vi "Sub03_PosTxt.vi"(8 "error in (no error)":errorcluster, 10 "String":string) -> (0 "error out":errorcluster, 3 "output cluster":T1, 5 "standard error":string, 7 "standard output":string)   [LabVIEW 2019]
panel:
  out "vi name":string
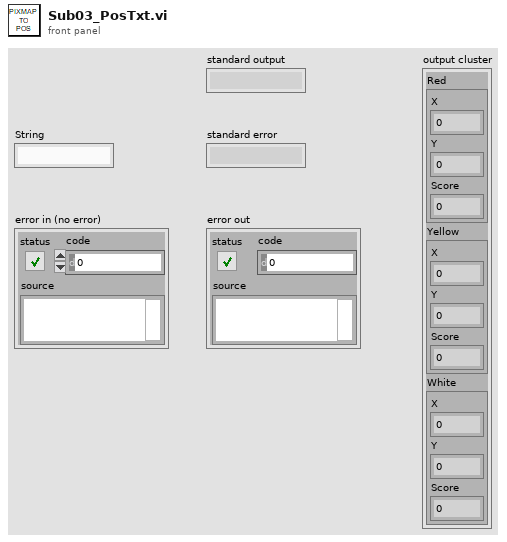
[diagram p1: front panel]
types:
  T1 = cluster{"Red":cluster{"X":u32, "Y":u32, "Score":u32}, "Yellow":cluster{"X":u32, "Y":u32, "Score":u32}, "White":cluster{"X":u32, "Y":u32, "Score":u32}}
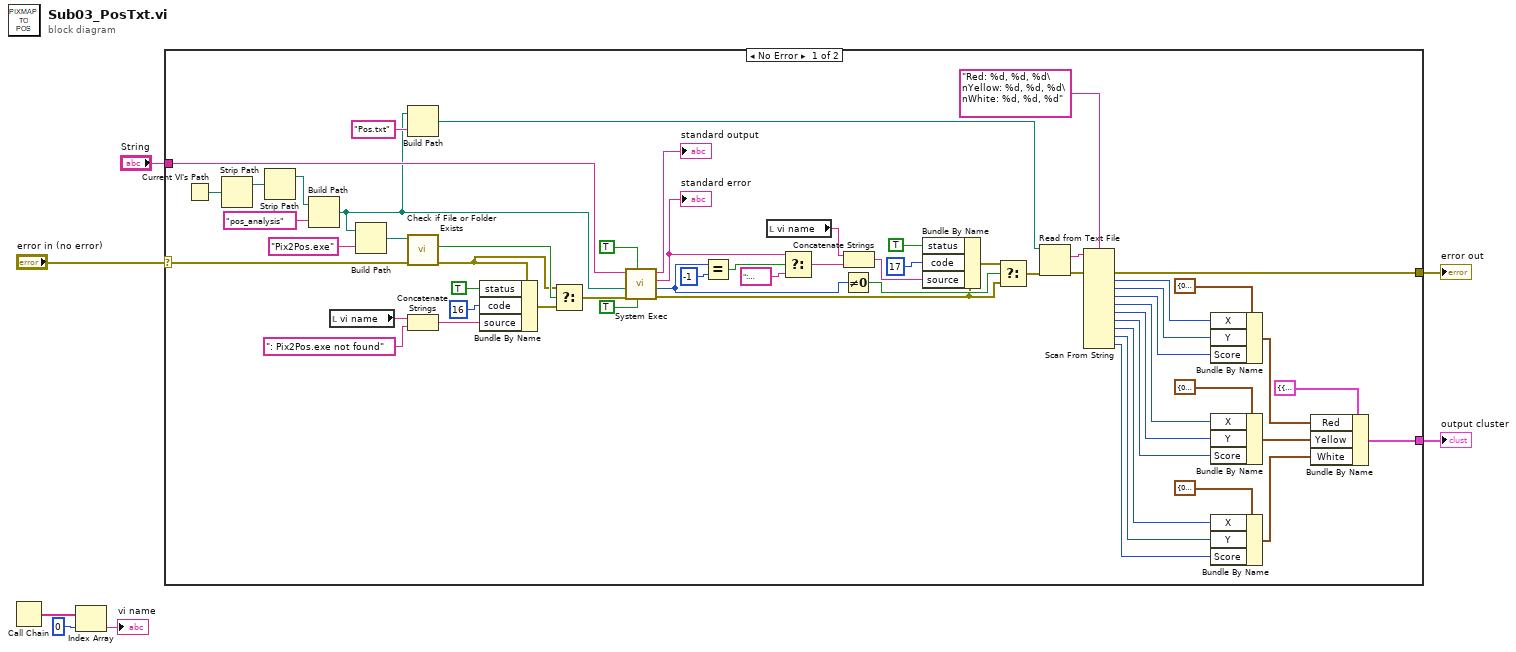
[diagram p0: block diagram]
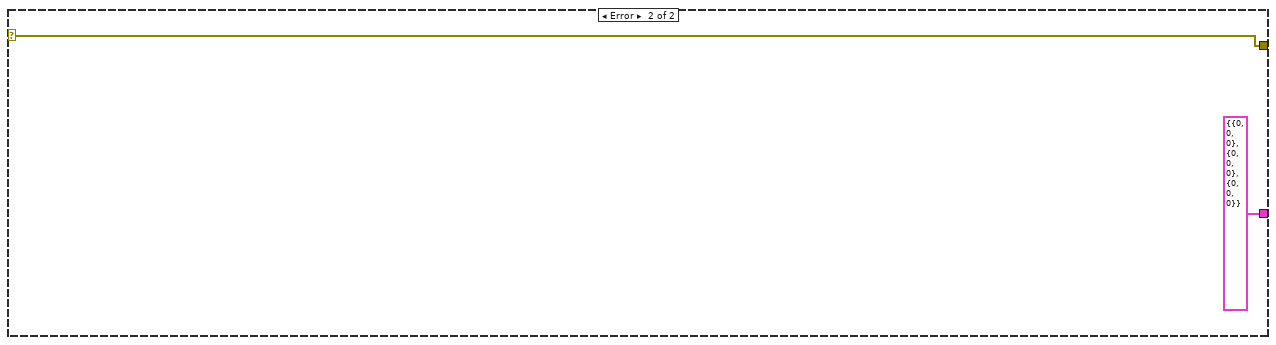
[diagram p2: hidden frame]
diagram:
  n1 = Call Chain() -> (call chain=w3:string[])
  n2 = Index Array(array=w3, index=0) -> (element=→"vi name":string)
  n3 = case shown="No Error" "error in (no error)" {
    selector: "error in (no error)" -> [w23 w66]
    tunnel: [w29 w66] -> w7
    tunnel: [w28 T1 {"Red"={"X"=0, "Y"=0, "Score"=0}, "Yellow"={"X"=0, "Y"=0, "Score"=0}, "White"={"X"=0, "Y"=0, "Score"=0}} ("output cluster")] -> w6
    tunnel: "String" -> [w27 _]
    frame No Error {
      n4 = Current VI's Path() -> (path=w30:path)
      n5 = Strip Path(path=w30) -> (stripped path=w11:path)  [unwired: 1 out]
      n6 = Strip Path(path=w11) -> (stripped path=w10:path)  [unwired: 1 out]
      n7 = Build Path(base path=w10, name or relative path="pos_analysis") -> (appended path=w9:path)
      n8 = local read "vi name"() -> (w13:string)
      n9 = Build Path(base path=w9, name or relative path="Pix2Pos.exe") -> (appended path=w26:path)
      n10 = Build Path(base path=w9, name or relative path="Pos.txt") -> (appended path=w60:path)
      n11 = call <vilib>:"Check if File or Folder Exists.vi"("error in (no error)"=w23, "path"=w26) -> ("error out"=w16:errorcluster, "file or folder exists?"=w24:bool)  [unwired: 7 in, 1 out]
      n12 = Concatenate Strings(w13, ": Pix2Pos.exe not found" ("string")) -> (w18:string)
      n13 = Bundle By Name(cluster=w16, "status"=TRUE, "code"=16, "source"=w18) -> (w17:errorcluster)
      n14 = Select(t=w16, s=w24, f=w17) -> (s? t:f=w22:errorcluster)
      n15 = call <vilib>:"System Exec.vi"("run minimized? (F)"=TRUE, "wait until completion? (T)"=TRUE, "error in (no error)"=w22, "working directory"=w9, "command line"=w27) -> ("error out"=w31:errorcluster, "return code"=w35:i32, "standard error"=w33:string, "standard output"=→"standard output":string)  [unwired: 3 in]
      "standard error" <- w33
      n16 = Equal?(x=w35, y=-1) -> (x = y?=w36:bool)
      n17 = local read "vi name"() -> (w12:string)
      n18 = Select(t=w33, s=w36, f=": unknown error during C execution") -> (s? t:f=w15:string)
      n19 = Not Equal To 0?(x=w35) -> (x != 0?=w37:bool)
      n20 = Concatenate Strings(w12, w15) -> (w14:string)
      n21 = Bundle By Name(cluster=w31, "status"=TRUE, "code"=17, "source"=w14) -> (w39:errorcluster)
      n22 = Select(t=w39, s=w37, f=w31) -> (s? t:f=w61:errorcluster)
      n23 = Read from Text File(file (use dialog)=w60, error in=w61) -> (text=w58:string, error out=w57:errorcluster)  [unwired: 2 in, 2 out]
      n24 = Scan From String(format string="Red: %d, %d, %d\nYellow: %d, %d, %d\nWhite: %d, %d, %d", input string=w58, error in=w57) -> (error out=w29:errorcluster, output 1=w56:i32, output 2=w55:i32, output 3=w54:i32, output 4=w53:i32, output 5=w52:i32, output 6=w51:i32, output 7=w49:i32, output 8=w48:i32, output 9=w47:i32)  [unwired: 10 in, 2 out]
      n25 = Bundle By Name(cluster=cluster{"X":u32, "Y":u32, "Score":u32} {"X"=0, "Y"=0, "Score"=0} ("Cluster"), "X"=w56, "Y"=w55, "Score"=w54) -> (w45:cluster{"X":u32, "Y":u32, "Score":u32})
      n26 = Bundle By Name(cluster=cluster{"X":u32, "Y":u32, "Score":u32} {"X"=0, "Y"=0, "Score"=0} ("Cluster"), "X"=w53, "Y"=w52, "Score"=w51) -> (w44:cluster{"X":u32, "Y":u32, "Score":u32})
      n27 = Bundle By Name(cluster=cluster{"X":u32, "Y":u32, "Score":u32} {"X"=0, "Y"=0, "Score"=0} ("Cluster"), "X"=w49, "Y"=w48, "Score"=w47) -> (w43:cluster{"X":u32, "Y":u32, "Score":u32})
      n28 = Bundle By Name(cluster=T1 {"Red"={"X"=0, "Y"=0, "Score"=0}, "Yellow"={"X"=0, "Y"=0, "Score"=0}, "White"={"X"=0, "Y"=0, "Score"=0}} ("output cluster"), "Red"=w45, "Yellow"=w44, "White"=w43) -> (w28:T1)
    }
    frame Error {
    }
  }
  "error out" <- w7
  "output cluster" <- w6
